vi "detect datatype.vi"(7 "error in (no error)":errorcluster, 10 "Ctl Refnum":refnum<vi>) -> (0 "error out":errorcluster, 2 "is supported?":bool, 3 "data type":T1)   [LabVIEW 2013]
uses:
  <vilib>/NI/Tag Bus/tag/Data Type.ctl
  <vilib>/Utility/VariantDataType/Type.ctl
  <vilib>/Utility/VariantDataType/VariantType.lvlib
  <vilib>/NI/Tag Bus/tag/tag descriptor.lvclass
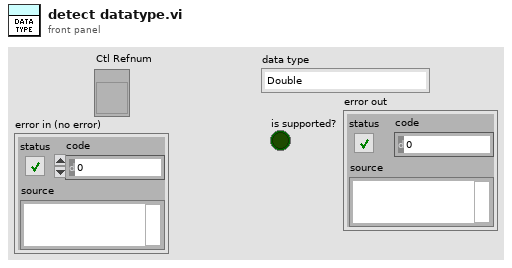
[diagram p1: front panel]
types:
  T1 = typedef "tag bus.lvlib/tag descriptor.lvclass/Data Type.ctl" = enum16{"Double", "Single", "I64", "I32", "I16", "I8", "U64", "U32", "U16", "U8", "Boolean", "String", "Array of Double", "Array of Single", "Array of I64", "Array of I32", "Array of I16", "Array of I8", "Array of U64", "Array of U32", "Array of U16", "Array of U8", "Array of Boolean", "Array of String"}
  T2 = typedef "VariantType.lvlib/Type.ctl" = enum8{"Invalid Type", "Void", "I8", "I16", "I32", "I64", "U8", "U16", "U32", "U64", "Single Float", "Double Float", "Extended Float", "Single Complex", "Double Complex", "Extended Complex", "Enum U8", "Enum U16", "Enum U32", "Enum U64", "Single Float With Unit", "Double Float With Unit", "Extended Float With Unit", "Single Complex with Unit", "Double Complex with Unit", "Extended Complex with Unit", "Boolean", "String", "Path", "Picture", "Tag", "Array", "Cluster", "Variant", "LV Variant", "Waveform", "Timestamp", "Digital Waveform", "Digital Data", "ExpressData", "Refnum", "External Data", "VI", "Poly VI", "LabVIEW Class Instance", "Fixed Point"}
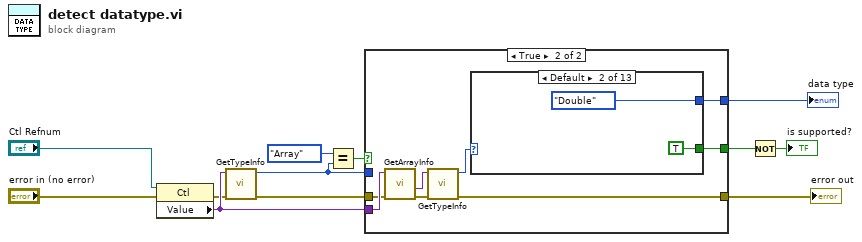
[diagram p0: block diagram]
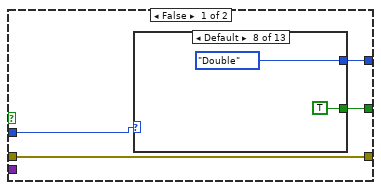
[diagram p2: hidden frame]
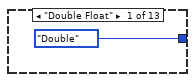
[diagram p3: hidden frame]
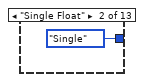
[diagram p4: hidden frame]
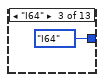
[diagram p5: hidden frame]
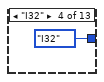
[diagram p6: hidden frame]
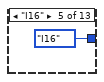
[diagram p7: hidden frame]
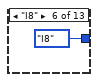
[diagram p8: hidden frame]
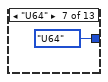
[diagram p9: hidden frame]
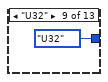
[diagram p10: hidden frame]
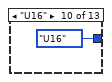
[diagram p11: hidden frame]
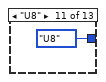
[diagram p12: hidden frame]
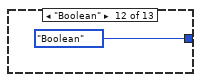
[diagram p13: hidden frame]
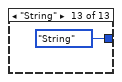
[diagram p14: hidden frame]
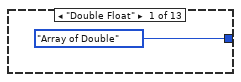
[diagram p15: hidden frame]
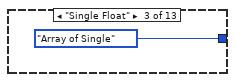
[diagram p16: hidden frame]
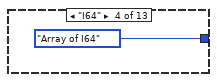
[diagram p17: hidden frame]
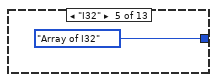
[diagram p18: hidden frame]
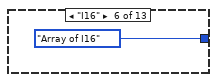
[diagram p19: hidden frame]
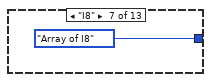
[diagram p20: hidden frame]
diagram:
  n1 = property class="Ctl"(reference="Ctl Refnum", error in="error in (no error)") -> (error out=w4:errorcluster, "Value"=w10:variant)  [unwired: 1 out]
  n2 = call <vilib>:"GetTypeInfo.vi"("error in (no error)"=w4, "Variant"=w10) -> ("error out"=w3:errorcluster, "Type Enum"=w8:T2)  [unwired: 5 in, 3 out]
  n3 = Equal?(x=Type."Array", y=w8) -> (x = y?=w11:bool)
  n4 = case shown="True" w11 {
    tunnel: w10 -> [_ w38]
    tunnel: [w15 w35] -> w9
    tunnel: w8 -> [w16 _]
    tunnel: [w14 w34] -> w6
    tunnel: w3 -> [w13 w33]
    tunnel: [w13 w31] -> w1
    frame False {
      n5 = case shown="Default" w16 {
        tunnel: [Data_Type."Double" ("data type") Data_Type."Single" ("data type") Data_Type."I64" ("data type") Data_Type."I32" ("data type") Data_Type."I16" ("data type") Data_Type."I8" ("data type") Data_Type."U64" ("data type") Data_Type."Double" ("data type") Data_Type."U32" ("data type") Data_Type."U16" ("data type") Data_Type."U8" ("data type") Data_Type."Boolean" ("data type") Data_Type."String" ("data type")] -> w15
        tunnel: [_ _ _ _ _ _ _ TRUE _ _ _ _ _] -> w14
        frame "Double Float" {
        }
        frame "Single Float" {
        }
        frame "I64" {
        }
        frame "I32" {
        }
        frame "I16" {
        }
        frame "I8" {
        }
        frame "U64" {
        }
        frame Default {
        }
        frame "U32" {
        }
        frame "U16" {
        }
        frame "U8" {
        }
        frame "Boolean" {
        }
        frame "String" {
        }
      }
    }
    frame True {
      n6 = call <vilib>:"GetArrayInfo.vi"("error in (no error)"=w33, "Variant"=w38) -> ("error out"=w32:errorcluster, "ArrayElement"=w37:variant)  [unwired: 6 in, 2 out]
      n7 = call <vilib>:"GetTypeInfo.vi"("error in (no error)"=w32, "Variant"=w37) -> ("error out"=w31:errorcluster, "Type Enum"=w36:T2)  [unwired: 5 in, 3 out]
      n8 = case shown="Default" w36 {
        tunnel: [Data_Type."Array of Double" ("data type") Data_Type."Double" ("data type") Data_Type."Array of Single" ("data type") Data_Type."Array of I64" ("data type") Data_Type."Array of I32" ("data type") Data_Type."Array of I16" ("data type") Data_Type."Array of I8" ("data type") Data_Type."Array of U64" ("data type") Data_Type."Array of U32" ("data type") Data_Type."Array of U16" ("data type") Data_Type."Array of U8" ("data type") Data_Type."Array of Boolean" ("data type") Data_Type."Array of String" ("data type")] -> w35
        tunnel: [_ TRUE _ _ _ _ _ _ _ _ _ _ _] -> w34
        frame "Double Float" {
        }
        frame Default {
        }
        frame "Single Float" {
        }
        frame "I64" {
        }
        frame "I32" {
        }
        frame "I16" {
        }
        frame "I8" {
        }
        frame "U64" {
        }
        frame "U32" {
        }
        frame "U16" {
        }
        frame "U8" {
        }
        frame "Boolean" {
        }
        frame "String" {
        }
      }
    }
  }
  "data type" <- w9
  "error out" <- w1
  n9 = Not(x=w6) -> (.not. x?=→"is supported?":bool)
